vi "Initialize Attributes Core.vi"(8 "error in (no error)":errorcluster, 10 "Attribute Data":variant, 11 "BNT_DAQmx_MCSV-Ctr2Freq in":refnum<class "BNT_DAQmx-MCSV-Ctr2Freq.lvclass">) -> (0 "error out":errorcluster, 2 "MandatoryParameters":cluster{"Parameter":string, "found?":bool}[](array[cluster]), 3 "BNT_DAQmx_MCSV-Ctr2Freq out":refnum<class "BNT_DAQmx-MCSV-Ctr2Freq.lvclass">)   [LabVIEW 2021, in "BNT_DAQmx.lvlib" / "BNT_DAQmx-MCSV-Ctr2Freq.lvclass"]
doc: "Initialize object attribute.\n\nUnique resources should be allocated elsewhere!"
uses:
  BNT_DAQmx-MCSV-Ctr2Freq.lvclass
  C:/Users/Holger/Documents/LVP/BNT/EQCR/Packages/CSPP_Core/Actors/CSPP_BaseActor/CSPP_BaseActor.lvclass
  CSPP_Core/Actors/CSPP_BaseActor/CSPP_BaseActor.lvclass/CSPP_BaseActor.ctl
  BNT_DAQmx-MCSV-Ctr2Freq.lvclass/BNT_DAQmx-MCSV-Ctr2Freq.ctl
  BNT_DAQmx-MCSV/BNT_DAQmx-MCSV.lvclass
  CSPP_Core/Classes/CSPP_BaseClasses/Factory/CSPP_Factory.lvclass
  CSPP_Core/Actors/CSPP_BaseActor/CSPP_BaseActor.lvclass
  CSPP_Core/Classes/CSPP_ProcessVariables/CSPP_ProcessVariables.lvlib
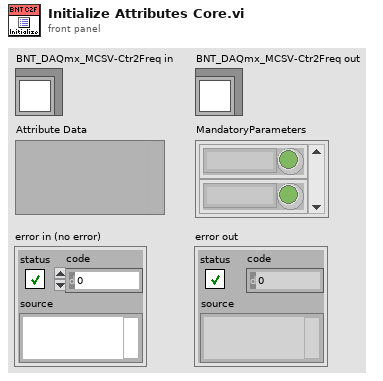
[diagram p1: front panel]
types:
  T1 = cluster{string, "Type Descriptor":string, string}
  T2 = cluster{"initial string":string, "Type Descriptor":string, string}
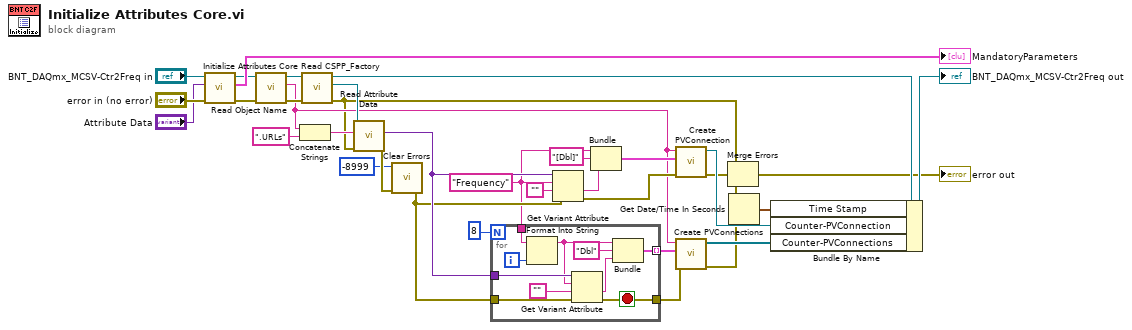
[diagram p0: block diagram]
diagram:
  w13 = "Frequency" ("initial string")
  n1 = call-parent "Initialize Attributes Core.vi"("error in (no error)"="error in (no error)", "Attribute Data"="Attribute Data", "BNT_DAQmx-MCSV in"="BNT_DAQmx_MCSV-Ctr2Freq in") -> ("error out"=w21:errorcluster, "MandatoryParameters"=→"MandatoryParameters":cluster{"Parameter":string, "found?":bool}[], "BNT_DAQmx-MCSV out"=w22:refnum<class "BNT_DAQmx-MCSV-Ctr2Freq.lvclass">)  [unwired: 6 in]
  n2 = call "Read Object Name.vi"("error in (no error)"=w21, "CSPP_BaseActor in"=w22) -> ("error out"=w20:errorcluster, "Object Name"=w6:string, "CSPP_BaseActor out"=w23:refnum<class "BNT_DAQmx-MCSV-Ctr2Freq.lvclass">)  [unwired: 7 in]
  n3 = Concatenate Strings(w6, ".URLs" ("string")) -> (w25:string)
  n4 = call "Read CSPP_Factory.vi"("error in (no error)"=w20, "CSPP_BaseActor in"=w23) -> ("error out"=w2:errorcluster, "CSPP_Factory"=w28:refnum<class "CSPP_Factory.lvclass">, "CSPP_BaseActor out"=w17:refnum<class "BNT_DAQmx-MCSV-Ctr2Freq.lvclass">)  [unwired: 7 in]
  n5 = call-dynamic "Read Attribute Data.vi"("error in (no error)"=w2, "Object Name"=w25, "CSPP_Factory in"=w28) -> ("error out"=w27:errorcluster, "Attribute Data"=w19:variant)  [unwired: 6 in, 1 out]
  n6 = call <vilib>:"Clear Errors.vi"("error in (no error)"=w27, "specific error code to clear (0: all)"=-8999) -> ("error out"=w18:errorcluster)  [unwired: 4 in, 1 out]
  n7 = for {
    N: 8 -> [_]
    tunnel: w19 -> [w43]
    tunnel: w18 -> [w42]
    tunnel: [w40] -> w5
    tunnel: w13 -> [w39]
    tunnel: [w35] -> w7 mode=indexing
    i -> [w41]
    stop <- w40 stop-if-true
    n8 = Format Into String(initial string=w39, w41) -> (resulting string=w38:string)  [unwired: 2 in, 1 out]
    n9 = Get Variant Attribute(Variant=w43, name=w38, default value (empty Variant)="", error in=w42) -> (value=w37:string, error out=w40:errorcluster)  [unwired: 2 out]
    n10 = Bundle(w38, "Type Descriptor"="Dbl", w37) -> (w35:T1)  [unwired: 1 in]
  }
  n11 = Get Variant Attribute(Variant=w19, name=w13, default value (empty Variant)="", error in=w18) -> (value=w11:string, error out=w8:errorcluster)  [unwired: 2 out]
  n12 = Bundle("initial string"=w13, "Type Descriptor"="[Dbl]", w11) -> (w10:T2)  [unwired: 1 in]
  n13 = call "Create PVConnection.vi"("Error In"=w8, "PV-Info"=w10, "Object Name"=w6) -> ("error out"=w3:errorcluster, "PVConnection"=w9:refnum<class "PVConnection.lvclass">)  [unwired: 7 in]
  n14 = call "Create PVConnections.vi"("Error In"=w5, "PV-Infos"=w7, "Object Name"=w6) -> ("error out"=w1:errorcluster, "PVConnections"=w4:refnum<class "PVConnection.lvclass">[])  [unwired: 7 in]
  n15 = Merge Errors(w2, w3, w1) -> (→"error out":errorcluster)
  n16 = Get Date/Time In Seconds() -> (seconds since 1Jan1904=w15:timestamp)
  n17 = Bundle By Name(cluster=w17, "Time Stamp"=w15, "Counter-PVConnection"=w9, "Counter-PVConnections"=w4) -> (→"BNT_DAQmx_MCSV-Ctr2Freq out":refnum<class "BNT_DAQmx-MCSV-Ctr2Freq.lvclass">)
